vi "Write Sensor Changes.vi"(7 "Index":i32, 9 "New":string, 10 "Old":string, 11 "Sensor DAO Class In":refnum<class "Sensor DAO Class.lvclass">) -> (3 "Sensor DAO Class Out":refnum<class "Sensor DAO Class.lvclass">)   [LabVIEW 2013]
uses:
  Sensor DAO Class.lvclass
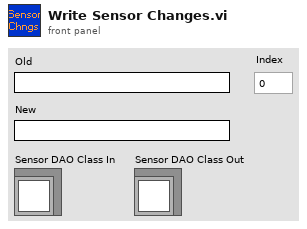
[diagram p1: front panel]
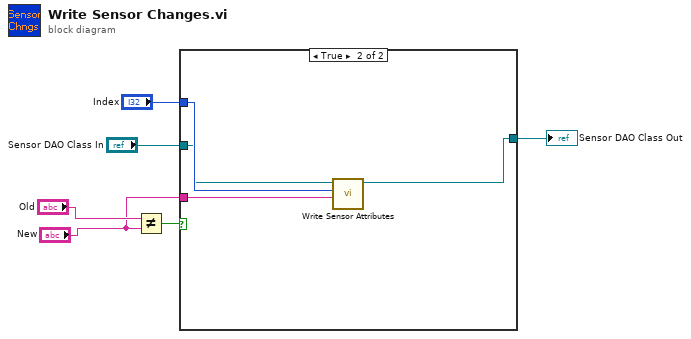
[diagram p0: block diagram]
diagram:
  n1 = Not Equal?(x="Old", y="New") -> (x != y?=w5:bool)
  n2 = case shown="True" w5 {
    tunnel: "Index" -> [_ w11]
    tunnel: "New" -> [_ w10]
    tunnel: "Sensor DAO Class In" -> [w7 w9]
    tunnel: [w7 w8] -> w1
    frame False {
    }
    frame True {
      n3 = call "Write Sensor Attributes.vi"("New"=w10, "Index"=w11, "Sensor DAO Class in"=w9) -> ("Sensor DAO Class out"=w8:refnum<class "Sensor DAO Class.lvclass">)  [unwired: 8 in]
    }
  }
  "Sensor DAO Class Out" <- w1
